vi "convert_to_json.vi"(8 "error in (no error)":errorcluster, 10 "data_set":variant, 11 "json_path":path) -> (0 "error out":errorcluster)   [LabVIEW 2015, in "lv-unit-conversion.lvlib"]
uses:
  lv-unit-conversion.lvlib
  _controls/data_set.ctl
  _controls/unit_set.ctl
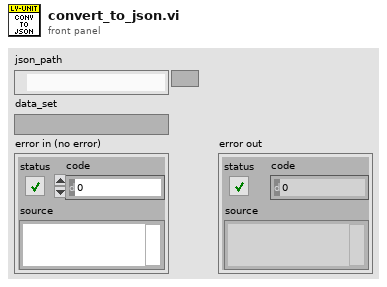
[diagram p1: front panel]
types:
  T1 = typedef "lv-unit-conversion.lvlib/data_set.ctl" = cluster{"unit_set":T2[]}
  T2 = typedef "lv-unit-conversion.lvlib/unit_set.ctl" = cluster{"symbol":string, "name":string, "dimension":string, "is_si_unit":bool, "category":string, "base_unit":string, "conversion_reference":string, "is_exact":bool, "a":dbl, "b":dbl, "c":dbl, "d":dbl, "underlying_def":string, "description":string}
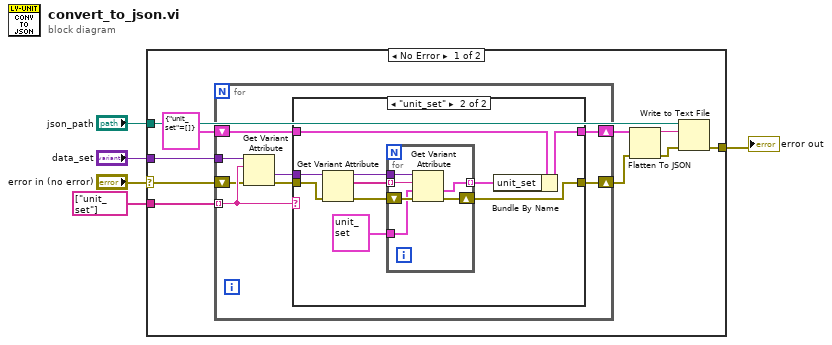
[diagram p0: block diagram]
diagram:
  n1 = case shown="No Error" "error in (no error)" {
    selector: "error in (no error)" -> [w13 w42]
    tunnel: "data_set" -> [w15 _]
    tunnel: string[] ["unit_set"] -> [w14 _]
    tunnel: [w7 w42] -> w2
    tunnel: "json_path" -> [w6 _]
    frame No Error {
      n2 = for {
        tunnel: w15 -> [w23]
        tunnel: w14 -> [w22] mode=indexing
        shift-right: [w16] -> w10
        shift-left: w13 -> [w21]
        shift-right: [w17] -> w11
        shift-left: T1 {"unit_set"=[]} -> [w18]
        n3 = Get Variant Attribute(Variant=w23, name=w22, error in=w21) -> (value=w20:variant, error out=w19:errorcluster)  [unwired: 1 in, 2 out]
        n4 = case shown="\"unit_set\"" w22 {
          tunnel: w20 -> [_ w35]
          tunnel: w19 -> [w24 w32]
          tunnel: w18 -> [w25 w29]
          tunnel: [w25 w28] -> w17
          tunnel: [w24 w26] -> w16
          frame Default {
          }
          frame "unit_set" {
            n5 = Get Variant Attribute(Variant=w35, error in=w32) -> (duplicate Variant=w33:variant, names=w34:string[], error out=w31:errorcluster)  [unwired: 2 in, 1 out]
            n6 = for {
              tunnel: w34 -> [w40] mode=indexing
              tunnel: w33 -> [w41]
              tunnel: T2 {"symbol"="", "name"="", "dimension"="", "is_si_unit"=FALSE, "category"="", "base_unit"="", "conversion_reference"="", "is_exact"=FALSE, "a"=0.0, "b"=0.0, "c"=0.0, "d"=0.0, "underlying_def"="", "description"=""} ("unit_set") -> [w38]
              tunnel: [w37] -> w27 mode=indexing
              shift-right: [w36] -> w26
              shift-left: w31 -> [w39]
              n7 = Get Variant Attribute(Variant=w41, name=w40, default value (empty Variant)=w38, error in=w39) -> (value=w37:T2, error out=w36:errorcluster)  [unwired: 2 out]
            }
            n8 = Bundle By Name(cluster=w29, "unit_set"=w27) -> (w28:T1)
          }
        }
      }
      n9 = Flatten To JSON(anything=w11, error in (no error)=w10) -> (JSON string=w9:string, 11:w8:errorcluster)  [unwired: 1 in]
      n10 = Write to Text File(file (use dialog)=w6, text=w9, error in=w8) -> (error out=w7:errorcluster)  [unwired: 1 in, 2 out]
    }
    frame Error {
    }
  }
  "error out" <- w2
